vi "calculate_derived_values_flexRIO.vi"(11 "scan specification":T2) -> (3 "derived values":T1)   [LabVIEW 2010]
uses:
  scan_specification_cluster_flexRIO.ctl
  derived_values_cluster_flexRIO.ctl
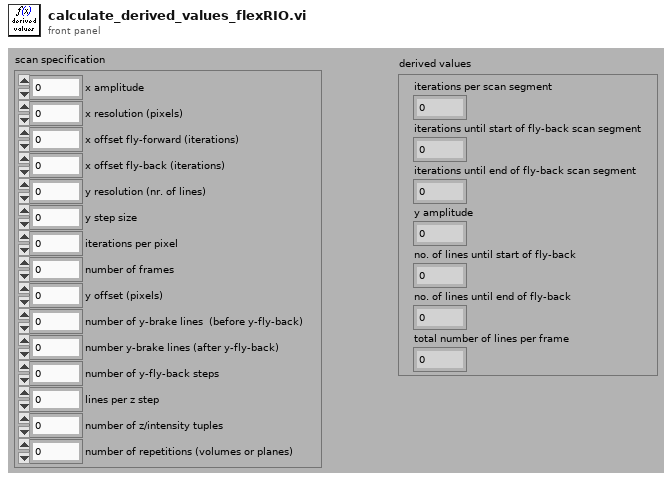
[diagram p1: front panel]
types:
  T1 = typedef "derived_values_cluster_flexRIO.ctl" = cluster{"iterations per scan segment":u16, "iterations until start of fly-back scan segment":u16, "iterations until end of fly-back scan segment":u16, "y amplitude":u16, "no. of lines until start of fly-back":u16, "no. of lines until end of fly-back":u16, "total number of lines per frame ":u16}
  T2 = typedef "scan_specification_cluster_flexRIO.ctl" = cluster{"x amplitude":u16, "x resolution (pixels)":u16, "x offset fly-forward (iterations)":u16, "x offset fly-back (iterations)":u16, "y resolution (nr. of lines)":u16, "y step size":u16, "iterations per pixel":u16, "number of frames":i32, "y offset (pixels)":u16, "number of y-brake lines  (before y-fly-back)":u16, "number y-brake lines (after y-fly-back)":u16, "number of y-fly-back steps":u16, "lines per z step":u16, "number of z/intensity tuples":u16, "number of repetitions (volumes or planes)":i32}
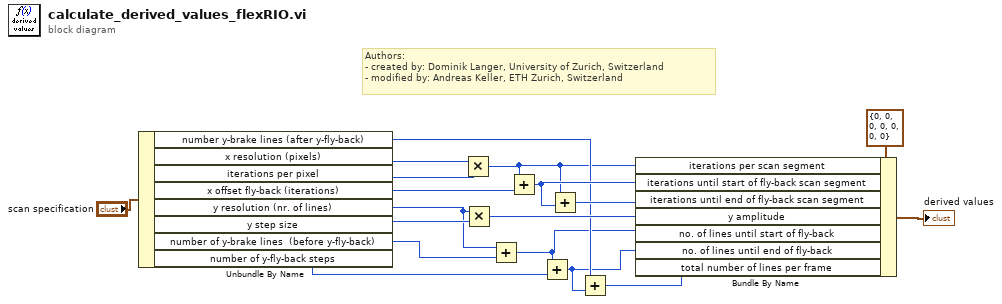
[diagram p0: block diagram]
diagram:
  # "Authors: \n- created by: Dominik Langer, University of Zurich, Switzerland\n- modified by: Andreas Keller, ETH Zurich, Switzerland"
  n1 = Unbundle By Name("scan specification") -> ("number y-brake lines (after y-fly-back)"=w7:u16, "x resolution (pixels)"=w16:u16, "iterations per pixel"=w15:u16, "x offset fly-back (iterations)"=w14:u16, "y resolution (nr. of lines)"=w9:u16, "y step size"=w11:u16, "number of y-brake lines  (before y-fly-back)"=w8:u16, "number of y-fly-back steps"=w4:u16)
  n2 = Multiply(x=w16, y=w15) -> (x*y=w3:u16)
  n3 = Multiply(x=w9, y=w11) -> (x*y=w10:u16)
  n4 = Add(x=w9, y=w8) -> (x+y=w5:u16)
  n5 = Add(x=w3, y=w14) -> (x+y=w13:u16)
  n6 = Add(x=w5, y=w4) -> (x+y=w6:u16)
  n7 = Add(x=w3, y=w13) -> (x+y=w12:u16)
  n8 = Add(x=w7, y=w6) -> (x+y=w2:u16)
  n9 = Bundle By Name(cluster=T1 {"iterations per scan segment"=0, "iterations until start of fly-back scan segment"=0, "iterations until end of fly-back scan segment"=0, "y amplitude"=0, "no. of lines until start of fly-back"=0, "no. of lines until end of fly-back"=0, "total number of lines per frame "=0} ("derived values"), "iterations per scan segment"=w3, "iterations until start of fly-back scan segment"=w13, "iterations until end of fly-back scan segment"=w12, "y amplitude"=w10, "no. of lines until start of fly-back"=w5, "no. of lines until end of fly-back"=w6, "total number of lines per frame"=w2) -> (→"derived values":T1)
